vi "Load_Write Status.vi"(10 "Load_Status":cluster{"kW":dbl}, 11 "Load in":refnum<class "Load.lvclass">) -> (3 "Load out":refnum<class "Load.lvclass">)   [LabVIEW 2015, in "Load.lvclass"]
uses:
  Load.lvclass
  Load.lvclass/Load.ctl
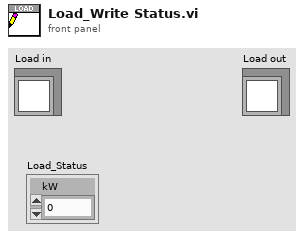
[diagram p1: front panel]
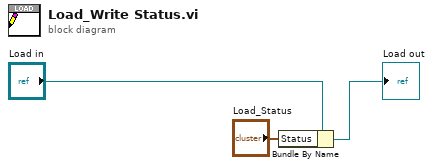
[diagram p0: block diagram]
diagram:
  n1 = Bundle By Name(cluster="Load in", "Status"="Load_Status") -> (→"Load out":refnum<class "Load.lvclass">)
